vi "FIR Filter PtByPt Multi-Channel861.vi"(7 "initialize":bool, 10 "Forward Coefficients":dbl[](array[numeric]), 11 "x":dbl[](array[numeric]) format="%0.2f") -> (0 "error":i32, 3 "Filtered x":dbl[](array[numeric]) format="%0.2f")   [LabVIEW 2014]
uses:
  <vilib>/Analysis/baseanly.llb/Vector x A.vi
  <vilib>/Analysis/NI_AALBase.lvlib
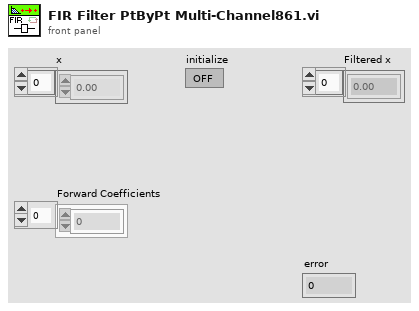
[diagram p1: front panel]
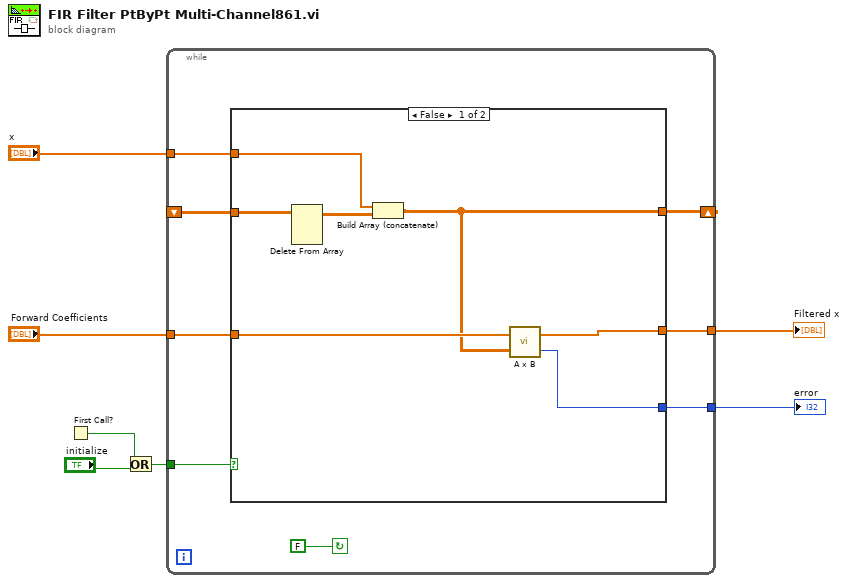
[diagram p0: block diagram]
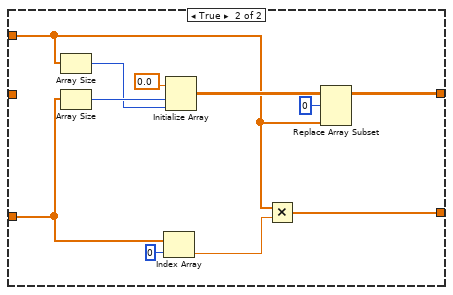
[diagram p2: hidden frame]
diagram:
  n1 = First Call?() -> (First Call?: T/F=w6:bool)
  n2 = Or(x=w6, y="initialize") -> (x .or. y?=w4:bool)
  n3 = while {
    tunnel: "x" -> [w11]
    shift-left: _ -> [w14]
    shift-right: [w13] -> _
    tunnel: "Forward Coefficients" -> [w12]
    tunnel: w4 -> [w10]
    tunnel: [w9] -> w2
    tunnel: [w8] -> w1
    stop <- FALSE continue-if-true
    n4 = case shown="False" w10 {
      tunnel: w12 -> [w19 w32]
      tunnel: w14 -> [w22 _]
      tunnel: [w17 w33] -> w9
      tunnel: [w18 w24] -> w13
      tunnel: w11 -> [w20 w25]
      tunnel: [w16 _] -> w8
      frame False {
        n5 = Delete From Array(array=w22) -> (array with subset deleted=w21:dbl[][])  [unwired: 3 in, 1 out]
        n6 = Build Array (concatenate)(w20, w21) -> (w18:dbl[][])
        n7 = call-poly <vilib>:"A x B.vi"("Matrix A"=w18, "Vector V'"=w19) -> ("error"=w16:i32, "V' x A"=w17:dbl[])
      }
      frame True {
        n8 = Array Size(array=w25) -> (size(s)=w27:i32)
        n9 = Array Size(array=w32) -> (size(s)=w28:i32)
        n10 = Index Array(array=w32, index=0 ("Index")) -> (element=w29:dbl)
        n11 = Initialize Array(0.0 ("Element Data"), w28, w27) -> (w26:dbl[][])
        n12 = Multiply(x=w25, y=w29) -> (x*y=w33:dbl[])
        n13 = Replace Array Subset(array=w26, new element=w25, index (row)=0) -> (w24:dbl[][])  [unwired: 1 in]
      }
    }
  }
  "error" <- w1
  "Filtered x" <- w2
